vi "UDFtoStr.vi"(3 "User Defined Functions":string) -> (1 "UDFString":string)   [LabVIEW 2013]
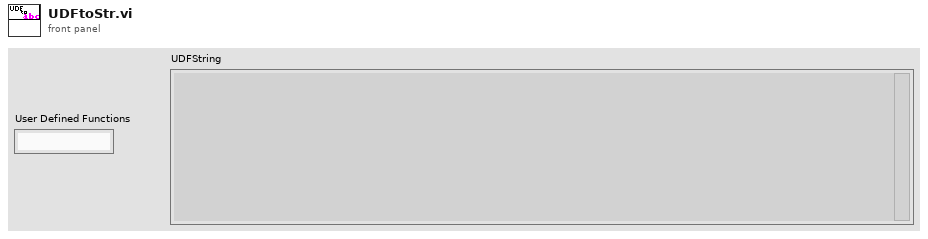
[diagram p1: front panel]
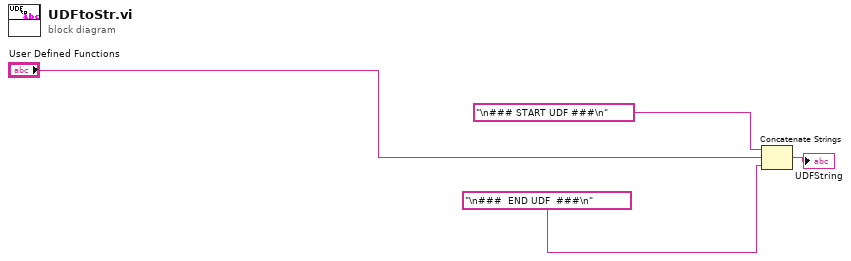
[diagram p0: block diagram]
diagram:
  n1 = Concatenate Strings("\n### START UDF ###\n" ("string"), "User Defined Functions", "\n###  END UDF  ###\n" ("string")) -> (→"UDFString":string)
